vi "Shutdown.vi"(8 "error in (no error)":errorcluster, 10 "Kill Now? (T)":bool=TRUE, 11 "BaseProducer in":refnum<class "BaseProducer.lvclass">) -> (0 "error out":errorcluster, 3 "BaseProducer out":refnum<class "BaseProducer.lvclass">)   [LabVIEW 2013, in "BaseProducer.lvclass"]
doc: "This method shuts the producer down, stopping IO tasks, closing data files, etc. This VI executes normally even if an error occurs before hand."
uses:
  BaseProducer.lvclass
  BaseProducer.lvclass/BaseProducer.ctl
  DbMeasurement/DbMeasurement.lvclass
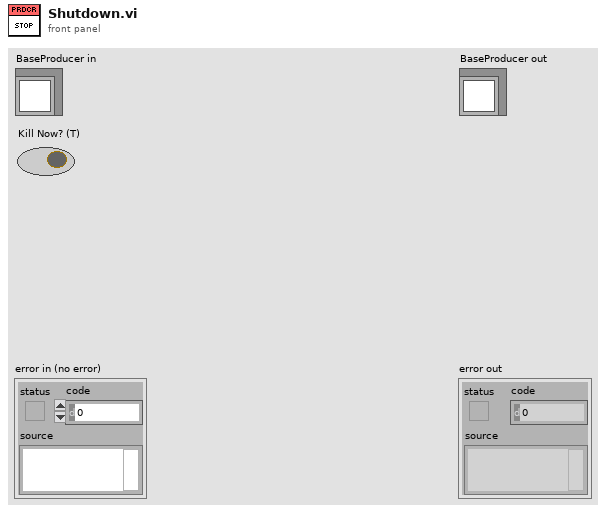
[diagram p1: front panel]
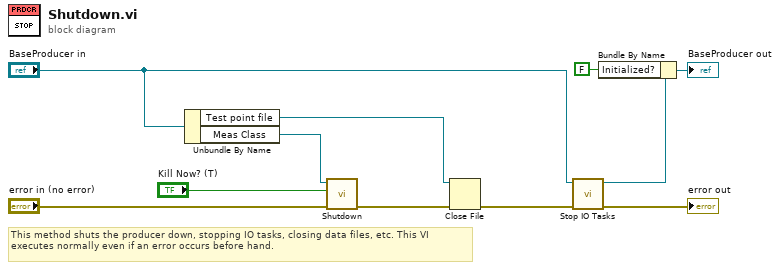
[diagram p0: block diagram]
diagram:
  # "This method shuts the producer down, stopping IO tasks, closing data files, etc. This VI executes normally even if an error occurs before hand."
  n1 = Unbundle By Name("BaseProducer in") -> ("Test point file"=w4:refnum<file>, "Meas Class"=w6:refnum<class "DbMeasurement.lvclass">)
  n2 = call "Shutdown.vi"("error in (no error)"="error in (no error)", "Kill Now? (T)"="Kill Now? (T)", "DbMeasurement in"=w6) -> ("error out"=w7:errorcluster)  [unwired: 7 in, 1 out]
  n3 = Close File(refnum=w4, error in=w7) -> (error out=w5:errorcluster)  [unwired: 1 out]
  n4 = call "Stop IO Tasks.vi"("error in (no error)"=w5, "BaseProducer in"="BaseProducer in") -> ("error out"=→"error out":errorcluster, "BaseProducer out"=w3:refnum<class "BaseProducer.lvclass">)  [unwired: 8 in]
  n5 = Bundle By Name(cluster=w3, "Initialized?"=FALSE) -> (→"BaseProducer out":refnum<class "BaseProducer.lvclass">)
